vi "WriteAdaptorr02.vi"(1 "error in (no error)":errorcluster, 2 "string to write":string="R5\n") -> (0 "error out":errorcluster)   [LabVIEW 2011]
doc: "The Basic Serial Read and Write example performs a Serial Port Read, a Serial Port Write, or a combination of these actions. The user selects the actions (read or write) on the front panel. If both are selected, the VI will write the data first, read data, and then close the VISA session that is opened to the port. This VI will wait until the specified number of bytes is received at the port or until a termination character is read.\n\nINSTRUCTIONS:\n1) Select the serial resource and configuration parameters (baud rate, data bits, parity, stop bits, flow control).\n2) Select the operations to be performed. \n3) Connect the serial port to your device. If no device is available, perform a loopback test by doing one of the following. Short pins 2 and 3 on a RS-232 cable or short pin 4 to pin 8 and pin 5 to pin 9 on a RS-485/422 cable. \n4) Run the VI to see the data read. (The \"read string\" will match the \"string to write\" if a loopback test was performed.)\n\nNote: The parameters set for the serial port must match the parameters of the connected instrument or device. In this example, the bytes to read parameter specifies the number of bytes that the serial port reads. If there were more bytes at the port than the number specified in bytes to read, those bytes would not be read. Also, if you specify to read more bytes than the number of bytes actually read, you might receive a timeout error message.\n\nOn the block diagram, the Configure Serial Port VI sets the configuration parameters. The front panel displays the controls used to configure the basic parameters, such as baud rate, data bits, and parity. Constants configure the other parameters the user probably does not need set. After the VISA Configure Serial Port VI opens the VISA session and configures the port, the VI passes the VISA resource name to other VIs that perform operations on that VISA resource. The VISA Write function sends a command to the serial device and the VISA Read function returns data based on the command. The VISA Close function then closes the reference to the serial device. It is important to close the reference; otherwise communication through with that port through protocols other than VISA might not be possible."
panel:
  out "concatenated string":string
  in  "Tab Control":enum32{"I/O", "AdapTorr"}(tab)
  in  "delay (ms)":u32=500
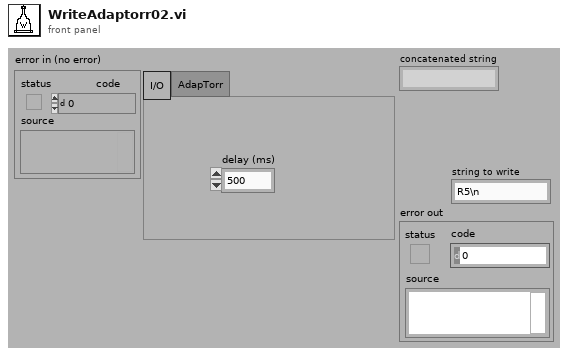
[diagram p1: front panel]
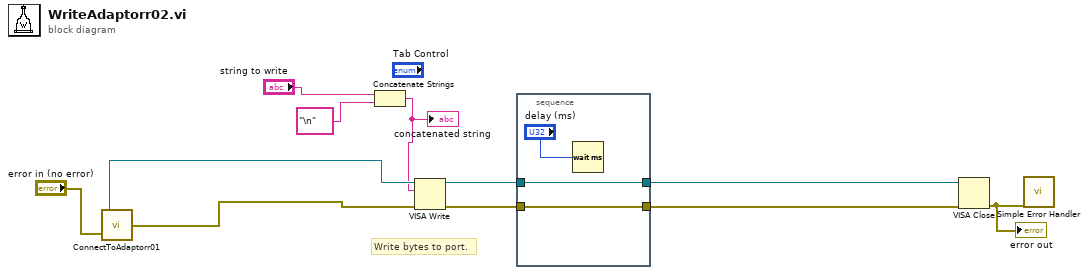
[diagram p0: block diagram]
diagram:
  # "Write bytes to port."
  n1 = call "ConnectToAdaptorr01.vi"("error in (no error)"="error in (no error)") -> ("error out"=w8:errorcluster, "VISA resource name out"=w5:refnum<visa-resource-name>)
  n2 = Concatenate Strings("string to write", "\n") -> (w1:string)
  "concatenated string" <- w1
  n3 = VISA Write(VISA resource name=w5, write buffer=w1, error in (no error)=w8) -> (VISA resource name out=w9:refnum<visa-resource-name>, error out=w10:errorcluster)  [unwired: 1 out]
  n4 = stacked-sequence {
    tunnel: w10 -> [w14]
    tunnel: [w14] -> w6
    tunnel: w9 -> [w13]
    tunnel: [w13] -> w7
    frame #0 {
      n5 = Wait (ms)(milliseconds to wait="delay (ms)") -> ()  [unwired: 1 out]
    }
  }
  n6 = VISA Close(VISA resource name=w7, error in (no error)=w6) -> (error out=w11:errorcluster)
  "error out" <- w11
  n7 = call <vilib>:"Simple Error Handler.vi"("error in (no error)"=w11) -> ()  [unwired: 1 in, 8 out]
